vi "Get Delay.vi"(8 "error in (no error)":errorcluster, 11 "VISA resource name":refnum<visa-resource-name>) -> (0 "error out":errorcluster, 2 "Delay (s)":dbl, 3 "VISA resource name out":refnum<visa-resource-name>)   [LabVIEW 2020, in "QuPMXdriver.lvlib"]
doc: "Returns the current enable delay."
uses:
  QuPMXdriver.lvlib
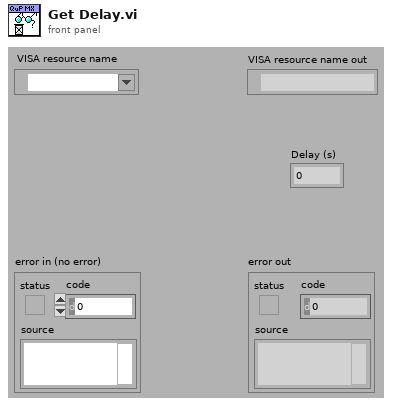
[diagram p1: front panel]
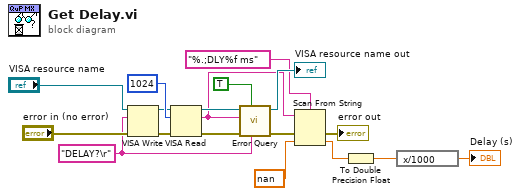
[diagram p0: block diagram]
diagram:
  w3 = "DELAY?\r"
  n1 = VISA Write(VISA resource name="VISA resource name", write buffer=w3, error in (no error)="error in (no error)") -> (VISA resource name out=w13:refnum<visa-resource-name>, error out=w2:errorcluster)  [unwired: 1 out]
  n2 = VISA Read(VISA resource name=w13, byte count=u32 1024, error in (no error)=w2) -> (VISA resource name out=w9:refnum<visa-resource-name>, read buffer=w4:string, error out=w8:errorcluster)  [unwired: 1 out]
  n3 = call "Error Query.vi"("Last command"=w3, "Ignore empty sequence? (T)"=TRUE, "error in (no error)"=w8, "Read buffer"=w4, "VISA resource name"=w9) -> ("error out"=w6:errorcluster, "VISA resource name out"=→"VISA resource name out":refnum<visa-resource-name>)  [unwired: 5 in]
  n4 = Scan From String(format string="%.;DLY%f ms", input string=w4, error in=w6, default 1=nan ("default value 1")) -> (error out=→"error out":errorcluster, output 1=w12:dbl)  [unwired: 1 in, 2 out]
  n5 = To Double Precision Float(number=w12) -> (double precision float=w11:dbl)
  n6 = expression code="x/1000"(w11) -> (→"Delay (s)":dbl)
